vi "myRIO v1.0 Build MUX Configuration AudioIn Block.vi"(11 "AudioIn (N Samples) Channels List":T4) -> (3 "Channel Reservation Info":T1)   [LabVIEW 2021]
uses:
  <vilib>/myRIO/Common/Instrument Driver Framework/myRIO v1.0/AudioIn Block/typedefs/AudioIn Block Channels List.ctl
  <vilib>/myRIO/Common/Instrument Driver Framework/myRIO v1.0/AudioIn Block/typedefs/AudioIn Block Channels Enum.ctl
  <vilib>/myRIO/Common/Instrument Driver Framework/myRIO v1.0/Resource Manager/typedefs/myRIO v1.0 Channel Reservation List.ctl
  <vilib>/myRIO/Common/Instrument Driver Framework/myRIO v1.0/Resource Manager/typedefs/myRIO v1.0 Channel Reservation Info.ctl
  <vilib>/myRIO/Common/Instrument Driver Framework/myRIO v1.0/Resource Manager/typedefs/myRIO v1.0 Connector List.ctl
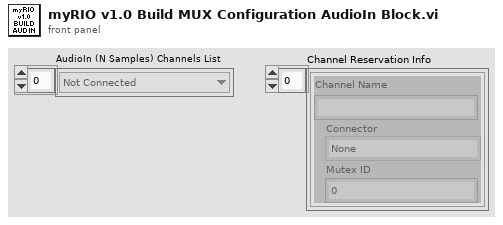
[diagram p1: front panel]
types:
  T1 = typedef "myRIO v1.0 Channel Reservation List.ctl" = T2[]
  T2 = typedef "myRIO v1.0 Channel Reservation Info.ctl" = cluster{"Channel Name":string, "Connector":T3, "Mutex ID":i32}
  T3 = typedef "myRIO v1.0 Connector List.ctl" = enum32{"None", "ConnectorA", "ConnectorB", "ConnectorC"}
  T4 = typedef "AudioIn Block Channels List.ctl" = T5[]
  T5 = typedef "AudioIn Block Channels Enum.ctl" = enum16{"Not Connected", "AudioIn/Left (N Samples)", "AudioIn/Right (N Samples)"}
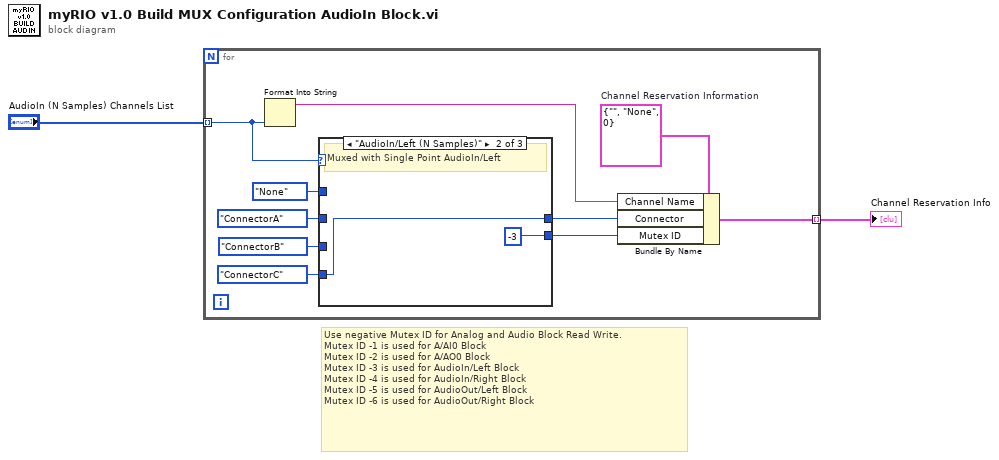
[diagram p0: block diagram]
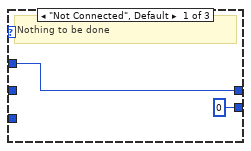
[diagram p2: hidden frame]
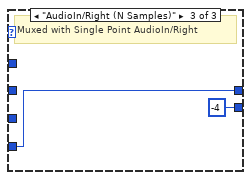
[diagram p3: hidden frame]
diagram:
  # "Use negative Mutex ID for Analog and Audio Block Read Write.\nMutex ID -1 is used for A/AI0 Block\nMutex ID -2 is used for A/AO0 Block\nMutex ID -3 is used for AudioIn/Left Block\nMutex ID -4 is used for AudioIn/Right Block\nMutex ID -5 is used for AudioOut/Left Block\nMutex ID -6 is used for AudioOut/Right Block"
  n1 = for {
    tunnel: "AudioIn (N Samples) Channels List" -> [w8] mode=indexing
    tunnel: [w9] -> w1 mode=indexing
    w12 = T2 {"Channel Name"="", "Connector"=enum."None", "Mutex ID"=0}  # Channel Reservation Information
    n2 = Format Into String(w8) -> (resulting string=w11:string)  [unwired: 3 in, 1 out]
    n3 = case shown="\"AudioIn/Left (N Samples)\"" w8 {
      tunnel: [0 ("Bit") -3 ("Bit") -4 ("Bit")] -> w10
      tunnel: myRIO_v1.0_Connector_List."None" ("Connector") -> [w14 _ _]
      tunnel: [w14 w15 w17] -> w6
      tunnel: myRIO_v1.0_Connector_List."ConnectorA" ("Connector") -> [_ _ _]
      tunnel: myRIO_v1.0_Connector_List."ConnectorB" ("Connector") -> [_ _ _]
      tunnel: myRIO_v1.0_Connector_List."ConnectorC" ("Connector") -> [_ w15 w17]
      frame "Not Connected", Default {
        # "Nothing to be done"
      }
      frame "AudioIn/Left (N Samples)" {
        # "Muxed with Single Point AudioIn/Left"
      }
      frame "AudioIn/Right (N Samples)" {
        # "Muxed with Single Point AudioIn/Right"
      }
    }
    n4 = Bundle By Name(cluster=w12, "Channel Name"=w11, "Connector"=w6, "Mutex ID"=w10) -> (w9:T2)
  }
  "Channel Reservation Info" <- w1
